vi "TTA_MATLAB_RX_Perform1RFIC1RxACPRTest.vi"(0 "Channel":string(combo), 1 "MXG VISA Resource In":refnum<visa-resource-name>, 2 "EXA VISA Resource":refnum<visa-resource-name>, 5 "Tx":string(combo), 11 "error in":errorcluster) -> (4 "ACPR\nResults":T1, 12 "MXG VISA Resource Out":refnum<visa-resource-name>, 13 "EXA VISA Resource Out":refnum<visa-resource-name>, 15 "error out":errorcluster)   [LabVIEW 2016]
uses:
  TTA_Globals/TTA_Global_Complete_Settings.vi
panel:
  out "RF Frequency":dbl[](array[numeric])
  out "ACPR Data":dbl[][](array[numeric])
  out "RFPAL PMU\nResults":dbl[][][](array[numeric])
  out "In Range?":bool[](array[boolean])
  out "Amp Max\nSpec (dBm)":dbl
  out "Amp Min\nSpec (dBm)":dbl
  out "IF Index":i32
  in  "PALLinearization Values":T2
  out "Tx#":i32
  out "CH#":i32
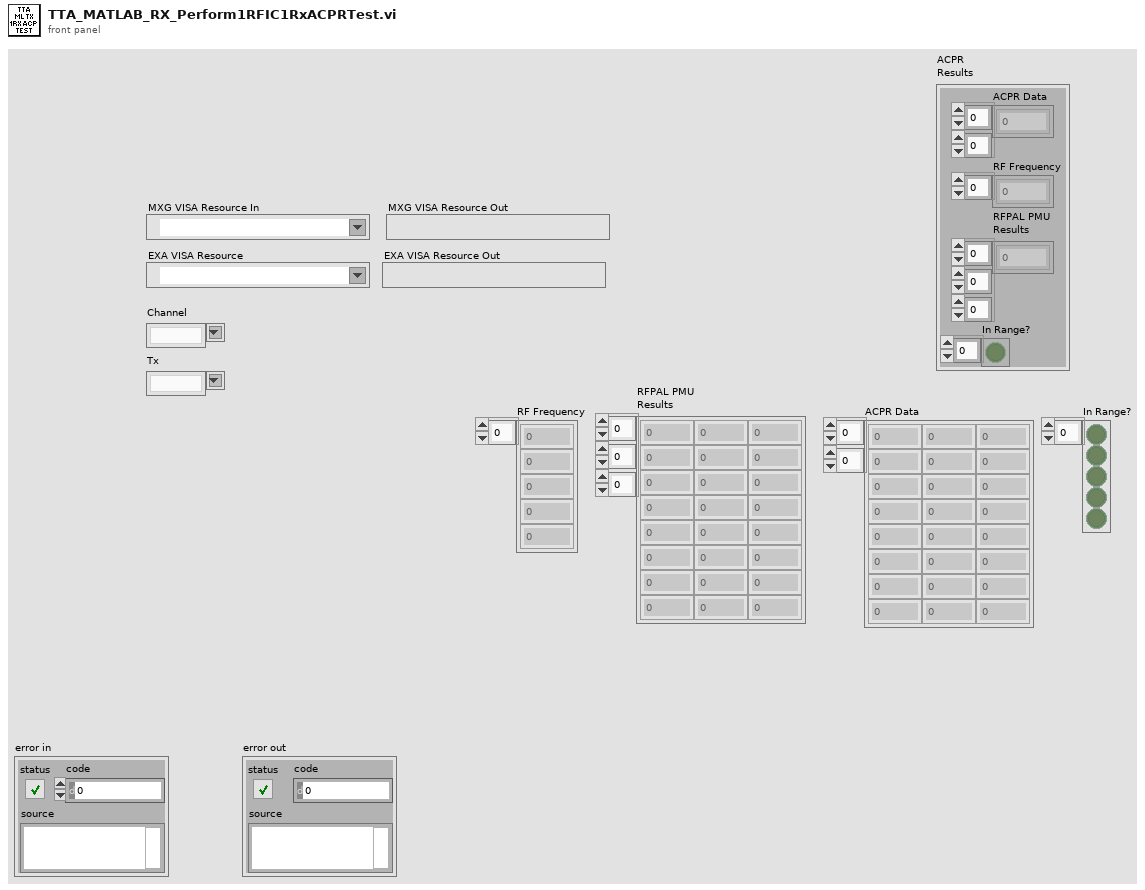
[diagram p1: front panel]
types:
  T1 = cluster{"ACPR Data":dbl[][], "RF Frequency":dbl[], "RFPAL PMU\nResults":dbl[][][], "In Range?":bool[]}
  T2 = cluster{"Tx IF Offsets":dbl[], "ACPR Filename":string, "Sampling Rate":dbl, "TxIF_Freq":dbl, "Power (dBm)":dbl, "IF Frequency Sweep (MHz)":dbl[], "BDSFreq":dbl, "Amplitude Range\nMax(dBm)":dbl, "Amplitude Range\nMin(dBm)":dbl, "CAL Amplitude\nIncrement(dB)":dbl, "CAL Amplitude\nDecrement (dB)":dbl, "Amplitude Least\nCriteria (dBm)":dbl}
  T3 = typedef "TTA_Control_Complete_Settings_Cluster.ctl" = cluster{"Brief Cluster":cluster{"STM Firmware File":string, "STM Firmware Address":string, "Required SW Version":string, "Template Used":string}, "Instrument Setting Cluster":cluster{"BDSFreq":dbl, "BDS Amp":dbl, "TxRFCal_Freq":dbl, "TxRFCal_Amp":dbl, "RxRFCal_Freq":dbl, "RxRFCal_Freq":dbl, "TxIF_Freq":dbl, "TxIF_Amp":dbl, "Tx_Output_Power_Signal_Freq":dbl, "Tx_ACPR_Signal_Freq":dbl, "Rx_RF_Freq":dbl, "Rx_RF_Amp":dbl, "Rx_Output_Power_Signal_Freq":dbl, "Rx_Output_Power_Sense_Freq":dbl}, "PAL Calibration\nInputs Cluster":cluster{"Amplitude Range\nMax(dBm)":dbl, "Amplitude Range\nMin(dBm)":dbl, "Amplitude Least\nCriteria (dBm)":dbl, "Frequency 1":dbl, "Frequency 2":dbl, "Frequency 3":dbl, "CAL Amplitude\nDecrement (dB)":dbl, "CAL Amplitude\nIncrement(dB)":dbl, "DownloadFile":string}, "TxOffset Cal Cluster":cluster{"Tx1 Offset (dB)":dbl, "Tx2 Offset (dB)":dbl, "Tx3 Offset (dB)":dbl, "Tx4 Offset (dB)":dbl, "Total RF Tx Loss (dB)":dbl}, "RxOffset Cal Cluster":cluster{"Rx1 Offset (dB)":dbl, "Rx2 Offset (dB)":dbl, "Rx3 Offset (dB)":dbl, "Rx4 Offset (dB)":dbl, "Total RF Rx Loss (dB)":dbl}, "TX Output Power Settings Cluster":cluster{"Frequency Sweep (MHz)":dbl[], "Sig Gen \nPower (dBm)":dbl, "Span (kHz)":dbl, "RBW (Hz)":dbl, "Ref Level (dBm)":dbl, "Low Power \nLimit":dbl, "High Power \nLimit":dbl, "DigAtt Max":dbl, "DigAtt Min":dbl}, "Tx ACPR Settings Cluster":cluster{"ACPR Filename":string, "Sampling Rate":dbl, "Power (dBm)":dbl, "IF Frequency Sweep (MHz)":dbl[], "State Name":string, "Mechanical\nAttenuation":dbl, "RefLevel Offset":dbl, "Amplitude Range\nMax (dBm)":dbl, "Amplitude Range\nMin (dBm)":dbl, "Cal Amp \nIncrement (dB)":dbl, "Cal Amp\nDecrement (dB)":dbl}, "Power Cal Cluster":cluster{"Power List (dBm)":dbl[], "Frequency (MHz)":dbl[], "Cal Decrement (dB)":dbl, "Cal Increment (dB)":dbl}, "Rx Received Power Settings Cluster":cluster{"Frequency Sweep (MHz)":dbl[], "Power (dBm)":dbl, "Span (kHz)":dbl, "RBW (Hz)":dbl, "Ref Level":dbl, "Low Power \nLimit (dBm)":dbl, "High Power\nLimit (dBm)":dbl}, "Tx Output Power Criteria Cluster":cluster{"CH1-TX1 \nMin":dbl, "CH1-TX1\nMax":dbl, "CH1-TXx3\nMin ":dbl, "CH1-TXx3\nMax":dbl, "CH2-TX1\nMin":dbl, "CH2-TX1\nMax":dbl, "CH2-TXx3\nMin":dbl, "CH2-TXx3\nMax":dbl}, "Tx ACPR Criteria Cluster":cluster{"Min Inband":dbl, "Max Close Outband":dbl, "Max Far Outband":dbl}, "Rx Output Power Criteria Cluster":cluster{"CH1-RX1 \nMin":dbl, "CH1-RX1 \nMax":dbl, "CH1-RXx3 \nMin":dbl, "CH1-RXx3\nMax":dbl, "CH2-RX1\nMin":dbl, "CH2-RX1\nMax":dbl, "CH2-RXx3\nMin":dbl, "CH2-RXx3\nMax":dbl}}
  T4 = cluster{"BDSFreq":dbl, "BDS Amp":dbl, "TxRFCal_Freq":dbl, "TxRFCal_Amp":dbl, "RxRFCal_Freq":dbl, "RxRFCal_Freq":dbl, "TxIF_Freq":dbl, "TxIF_Amp":dbl, "Tx_Output_Power_Signal_Freq":dbl, "Tx_ACPR_Signal_Freq":dbl, "Rx_RF_Freq":dbl, "Rx_RF_Amp":dbl, "Rx_Output_Power_Signal_Freq":dbl, "Rx_Output_Power_Sense_Freq":dbl}
  T5 = cluster{"Amplitude Range\nMax(dBm)":dbl, "Amplitude Range\nMin(dBm)":dbl, "Amplitude Least\nCriteria (dBm)":dbl, "Frequency 1":dbl, "Frequency 2":dbl, "Frequency 3":dbl, "CAL Amplitude\nDecrement (dB)":dbl, "CAL Amplitude\nIncrement(dB)":dbl, "DownloadFile":string}
  T6 = cluster{"Tx1 Offset (dB)":dbl, "Tx2 Offset (dB)":dbl, "Tx3 Offset (dB)":dbl, "Tx4 Offset (dB)":dbl, "Total RF Tx Loss (dB)":dbl}
  T7 = cluster{"ACPR Filename":string, "Sampling Rate":dbl, "Power (dBm)":dbl, "IF Frequency Sweep (MHz)":dbl[], "State Name":string, "Mechanical\nAttenuation":dbl, "RefLevel Offset":dbl, "Amplitude Range\nMax (dBm)":dbl, "Amplitude Range\nMin (dBm)":dbl, "Cal Amp \nIncrement (dB)":dbl, "Cal Amp\nDecrement (dB)":dbl}
  T8 = cluster{"CH1-TX1 \nMin":dbl, "CH1-TX1\nMax":dbl, "CH1-TXx3\nMin ":dbl, "CH1-TXx3\nMax":dbl, "CH2-TX1\nMin":dbl, "CH2-TX1\nMax":dbl, "CH2-TXx3\nMin":dbl, "CH2-TXx3\nMax":dbl}
  T9 = cluster{"Min Inband":dbl, "Max Close Outband":dbl, "Max Far Outband":dbl}
  T10 = cluster{"Amplitude Range\nMax (dBm)":dbl, "Amplitude Range\nMin (dBm)":dbl, "Cal Amp\nDecrement (dB)":dbl, "Cal Amp \nIncrement (dB)":dbl, "Amplitude Least\nCriteria (dBm)":dbl}
  T11 = enum16{"TX1", "TX2", "TX3", "TX4", "TXx3", "TXx4", "RX1", "RX2", "RX3", "RX4", "RXx3", "RXx4", "RFCal"}
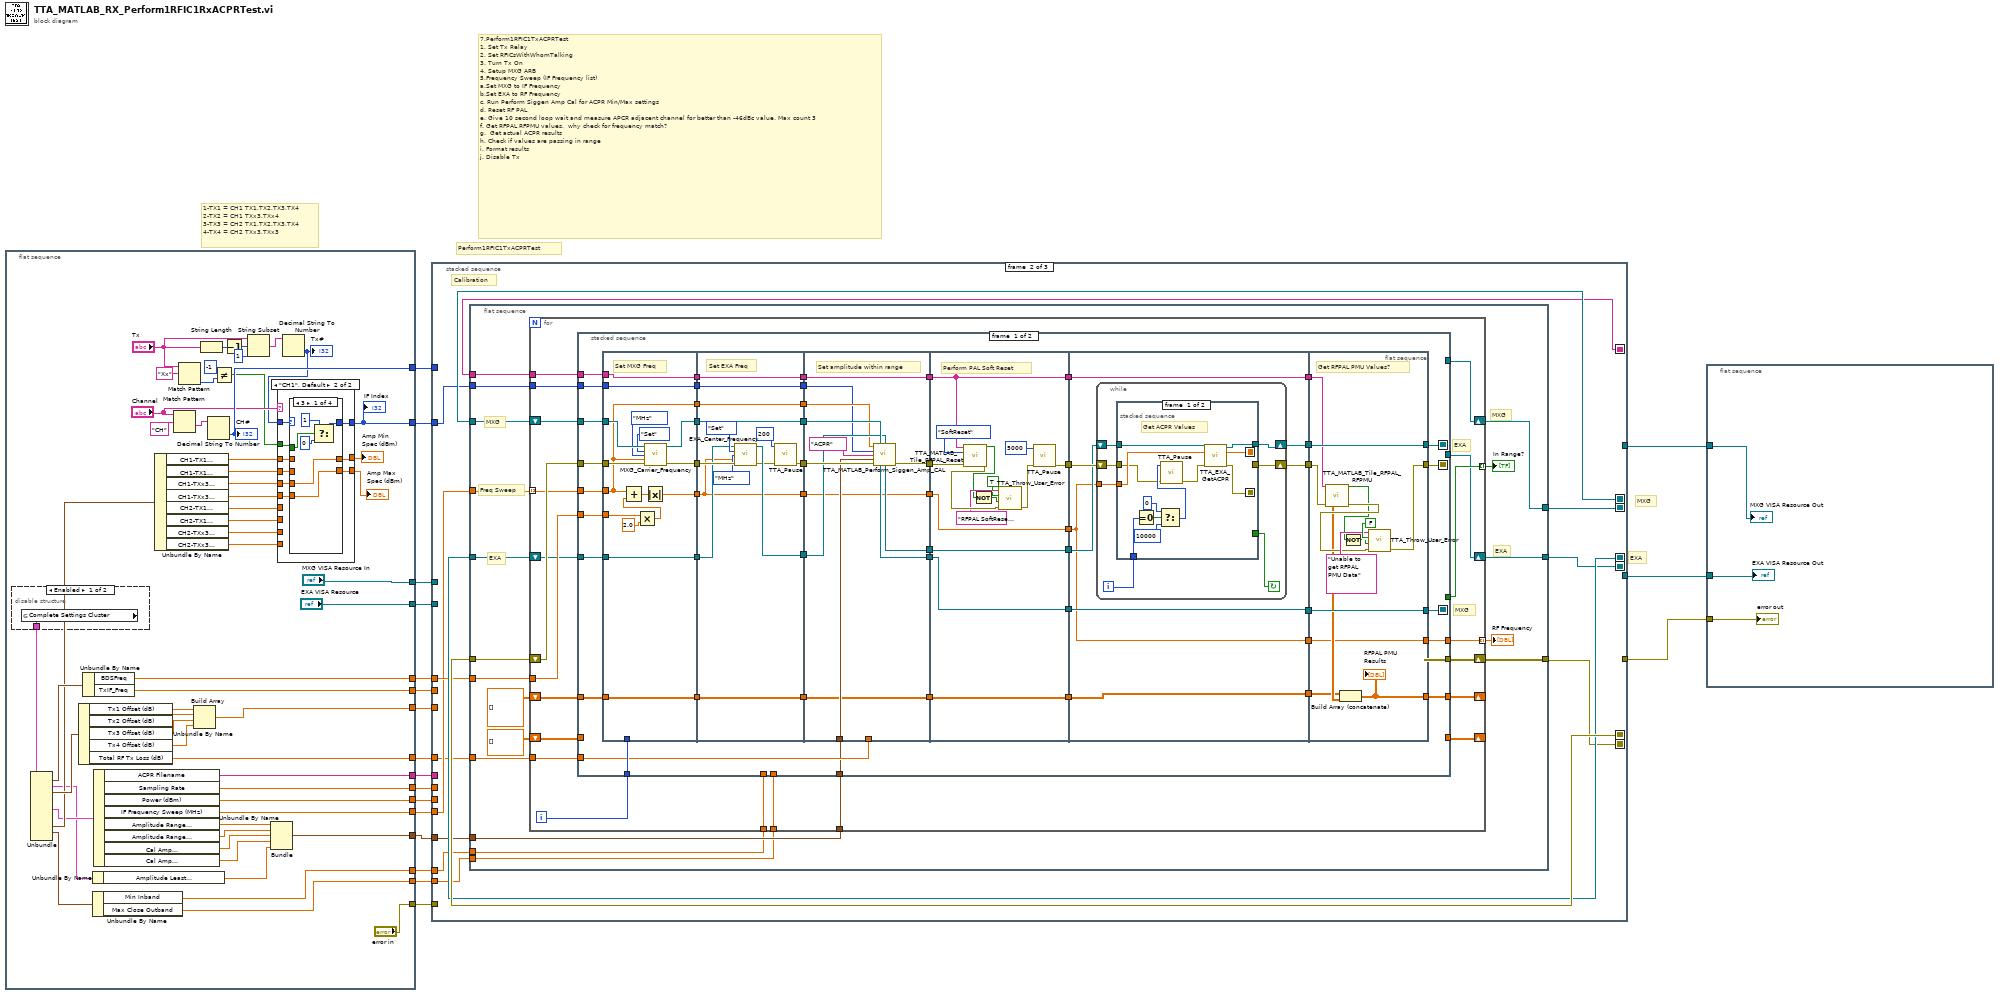
[diagram p0: block diagram]
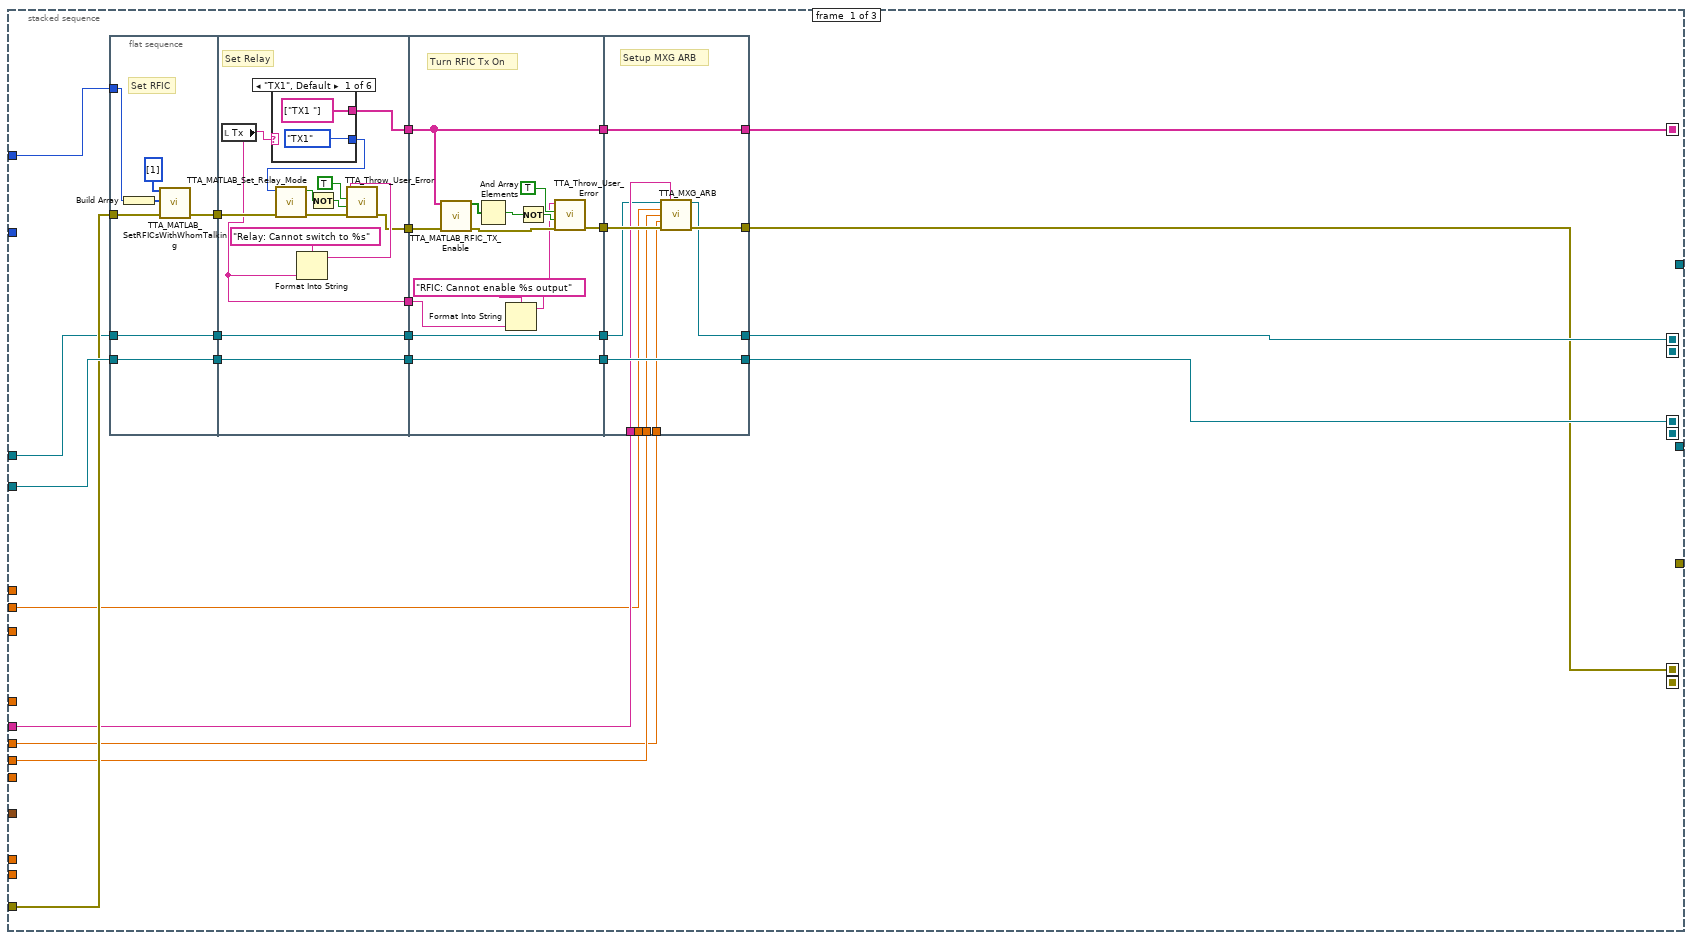
[diagram p2: hidden frame]
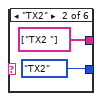
[diagram p3: hidden frame]
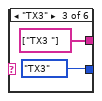
[diagram p4: hidden frame]
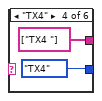
[diagram p5: hidden frame]
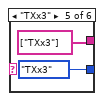
[diagram p6: hidden frame]
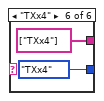
[diagram p7: hidden frame]
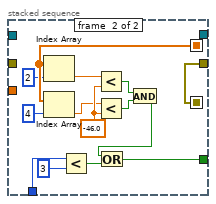
[diagram p8: hidden frame]
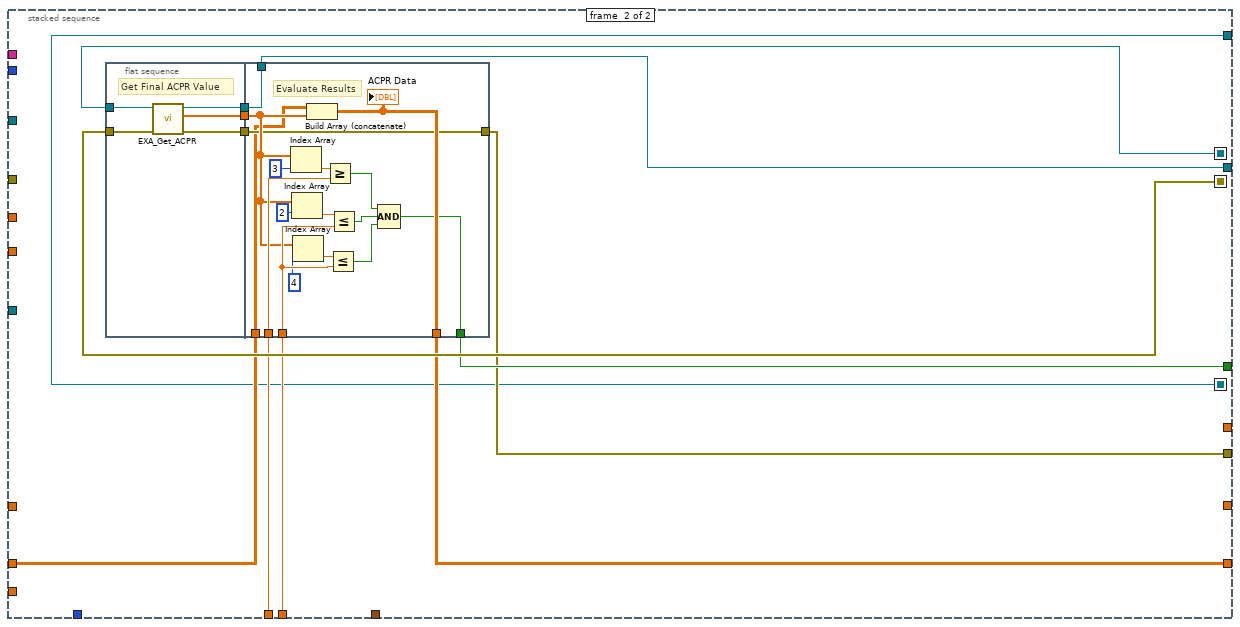
[diagram p9: hidden frame]
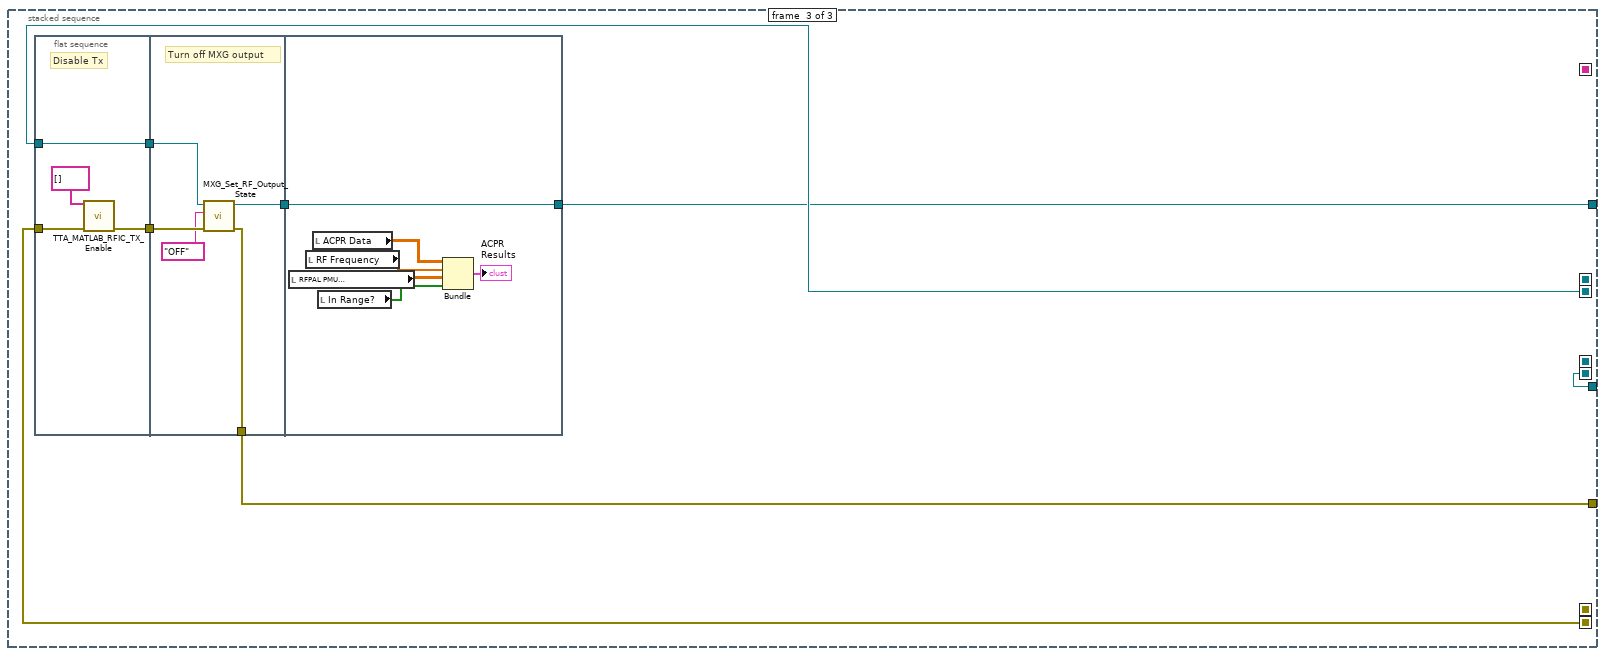
[diagram p10: hidden frame]
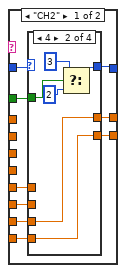
[diagram p11: hidden frame]
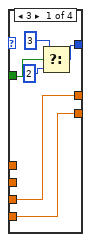
[diagram p12: hidden frame]
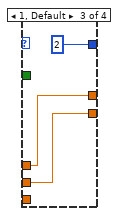
[diagram p13: hidden frame]
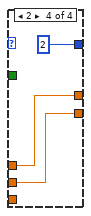
[diagram p14: hidden frame]
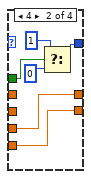
[diagram p15: hidden frame]
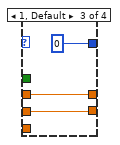
[diagram p16: hidden frame]
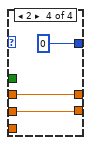
[diagram p17: hidden frame]
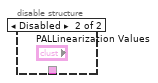
[diagram p18: hidden frame]
diagram:
  # "Perform1RFIC1TxACPRTest"
  # "7.Perform1RFIC1TxACPRTest\n1. Set Tx Relay\n2. Set RFICsWithWhomTalking\n3. Turn Tx On\n4. Setup MXG ARB\n5.Frequency Sweep (IF Frequency list)\na.Set MXG to IF Frequency\nb.Set EXA to RF Frequency\nc. Run Perform Siggen Amp Cal for ACPR Min/Max settings\nd. Reset RF PAL\ne. Give 10 second loop wait and measure APCR adjacent channel for better than -46dBc value. Max count 3\nf. Get RFPAL RFPMU values.  why check for frequency match?\ng.  Get actual ACPR results\nh. Check if values are passing in range\ni. Format results\nj. Disable Tx"
  # "1-TX1 = CH1 TX1,TX2,TX3,TX4\n2-TX2 = CH1 TXx3,TXx4\n3-TX3 = CH2 TX1,TX2,TX3,TX4\n4-TX4 = CH2 TXx3,TXx3"
  # "EXA"
  # "MXG"
  n1 = flat-sequence {
    tunnel: ["error in"] -> w19
    tunnel: ["MXG VISA Resource In"] -> w17
    tunnel: ["EXA VISA Resource"] -> w16
    tunnel: [w69] -> w18
    tunnel: [w55] -> w13
    tunnel: [w56] -> w12
    tunnel: [w61] -> w11
    tunnel: [w47] -> w10
    tunnel: [w33] -> w9
    tunnel: [w46] -> w8
    tunnel: [w32] -> w6
    tunnel: [w31] -> w5
    tunnel: [w30] -> w4
    tunnel: [w23] -> w3
    tunnel: [w21] -> w2
    tunnel: [w20] -> w1
    frame #0 {
      n2 = disable-structure shown="Enabled" {
        disable-tunnel: [w129 _] -> w64
        frame Enabled {
          n3 = global read "TTA_Global_Complete_Settings.vi" "Complete Settings Cluster"() -> (w129:T3)
        }
        frame Disabled {
        }
      }
      n4 = Unbundle(w64) -> ("Instrument Setting Cluster"=w63:T4, "PAL Calibration\nInputs Cluster"=w29:T5, "TxOffset Cal Cluster"=w62:T6, "Tx ACPR Settings Cluster"=w34:T7, "Tx Output Power Criteria Cluster"=w45:T8, "Tx ACPR Criteria Cluster"=w22:T9)  [unwired: 6 out]
      n5 = Unbundle By Name(w62) -> ("Tx1 Offset (dB)"=w60:dbl, "Tx2 Offset (dB)"=w59:dbl, "Tx3 Offset (dB)"=w58:dbl, "Tx4 Offset (dB)"=w57:dbl, "Total RF Tx Loss (dB)"=w46:dbl)
      n6 = Unbundle By Name(w63) -> ("BDSFreq"=w61:dbl, "TxIF_Freq"=w55:dbl)
      n7 = Unbundle By Name(w29) -> ("Amplitude Least\nCriteria (dBm)"=w24:dbl)
      n8 = Unbundle By Name(w22) -> ("Min Inband"=w21:dbl, "Max Close Outband"=w20:dbl)
      n9 = Unbundle By Name(w34) -> ("ACPR Filename"=w32:string, "Sampling Rate"=w30:dbl, "Power (dBm)"=w31:dbl, "IF Frequency Sweep (MHz)"=w33:dbl[], "Amplitude Range\nMax (dBm)"=w28:dbl, "Amplitude Range\nMin (dBm)"=w27:dbl, "Cal Amp\nDecrement (dB)"=w26:dbl, "Cal Amp \nIncrement (dB)"=w25:dbl)
      n10 = Unbundle By Name(w45) -> ("CH1-TX1 \nMin"=w44:dbl, "CH1-TX1\nMax"=w43:dbl, "CH1-TXx3\nMin"=w42:dbl, "CH1-TXx3\nMax"=w41:dbl, "CH2-TX1\nMin"=w40:dbl, "CH2-TX1\nMax"=w39:dbl, "CH2-TXx3\nMin"=w38:dbl, "CH2-TXx3\nMax"=w37:dbl)
      n11 = Match Pattern(string="Channel", regular expression="CH") -> (after substring=w70:string)  [unwired: 1 in, 3 out]
      n12 = Match Pattern(string="Tx", regular expression="Xx") -> (offset past match=w50:i32)  [unwired: 1 in, 3 out]
      n13 = Build Array(w60, w59, w58, w57) -> (w56:dbl[])
      n14 = String Length(string="Tx") -> (length=w68:i32)
      n15 = Decimal String To Number(string=w70) -> (number=w69:i32)  [unwired: 2 in, 1 out]
      "CH#" <- w69
      n16 = Not Equal?(x=-1, y=w50) -> (x != y?=w48:bool)
      n17 = Decrement(x=w68) -> (x-1=w67:i32)
      n18 = String Subset(string="Tx", offset (0)=w67, length (rest)=1 ("length (rest)")) -> (substring=w65:string)
      n19 = Bundle("Amplitude Range\nMax (dBm)"=w28, "Amplitude Range\nMin (dBm)"=w27, "Cal Amp\nDecrement (dB)"=w26, "Cal Amp \nIncrement (dB)"=w25, "Amplitude Least\nCriteria (dBm)"=w24) -> (w23:T10)  [unwired: 1 in]
      n20 = Decimal String To Number(string=w65) -> (number=w53:i32)  [unwired: 2 in, 1 out]
      "Tx#" <- w53
      n21 = case shown="\"CH1\", Default" "Channel" {
        tunnel: w53 -> [w82 w110]
        tunnel: [w83 w109] -> w47
        tunnel: w48 -> [w81 w108]
        tunnel: w44 -> [_ w107]
        tunnel: w43 -> [_ w106]
        tunnel: w42 -> [_ w105]
        tunnel: w41 -> [_ w104]
        tunnel: w40 -> [w80 _]
        tunnel: w39 -> [w79 _]
        tunnel: w38 -> [w78 _]
        tunnel: w37 -> [w77 _]
        tunnel: [w76 w103] -> w36
        tunnel: [w75 w102] -> w35
        frame "CH2" {
          n22 = case shown="4" w82 {
            tunnel: [w87 w93 2 2] -> w83
            tunnel: w81 -> [w86 w92 _ _]
            tunnel: w80 -> [_ _ w97 w100]
            tunnel: [w85 w91 w97 w100] -> w76
            tunnel: w79 -> [_ _ w96 w99]
            tunnel: [w84 w90 w96 w99] -> w75
            tunnel: w78 -> [w85 w91 _ _]
            tunnel: w77 -> [w84 w90 _ _]
            frame 3 {
              n23 = Select(t=3, s=w86, f=2) -> (s? t:f=w87:i32)
            }
            frame 4 {
              n24 = Select(t=3, s=w92, f=2) -> (s? t:f=w93:i32)
            }
            frame 1, Default {
            }
            frame 2 {
            }
          }
        }
        frame "CH1", Default {
          n25 = case shown="3" w110 {
            tunnel: [w114 w120 0 0] -> w109
            tunnel: w108 -> [w113 w119 _ _]
            tunnel: [w112 w118 w124 w127] -> w103
            tunnel: w107 -> [_ _ w124 w127]
            tunnel: [w111 w117 w123 w126] -> w102
            tunnel: w106 -> [_ _ w123 w126]
            tunnel: w105 -> [w112 w118 _ _]
            tunnel: w104 -> [w111 w117 _ _]
            frame 3 {
              n26 = Select(t=1, s=w113, f=0) -> (s? t:f=w114:i32)
            }
            frame 4 {
              n27 = Select(t=1, s=w119, f=0) -> (s? t:f=w120:i32)
            }
            frame 1, Default {
            }
            frame 2 {
            }
          }
        }
      }
      "IF Index" <- w47
      "Amp Min\nSpec (dBm)" <- w36
      "Amp Max\nSpec (dBm)" <- w35
    }
  }
  n28 = stacked-sequence {
    seq-local: [w130 _ _] -> [_ w222 _]
    seq-local: [w142 _ _] -> [_ w219 _]
    seq-local: [w143 _ _] -> [_ w221 _]
    seq-local: [_ w216 _] -> [_ _ w460]
    seq-local: [_ w214 _] -> [_ _ w466]
    seq-local: [_ w215 _] -> [_ _ w463]
    seq-local: [w131 _ _] -> [_ w211 _]
    tunnel: w19 -> [w141 _ _]
    tunnel: w18 -> [w153 _ _]
    tunnel: w17 -> [w140 _ _]
    tunnel: w16 -> [w151 _ _]
    tunnel: [_ _ w463] -> w15
    tunnel: [_ _ w462] -> w14
    tunnel: w13 -> [w134 _ _]
    tunnel: w12 -> [_ _ _]
    tunnel: w11 -> [_ w220 _]
    tunnel: w10 -> [_ w213 _]
    tunnel: w9 -> [_ w218 _]
    tunnel: w8 -> [_ w217 _]
    tunnel: [_ _ w464] -> w7
    tunnel: w6 -> [w135 _ _]
    tunnel: w5 -> [w133 _ _]
    tunnel: w4 -> [w132 _ _]
    tunnel: w3 -> [_ w212 _]
    tunnel: w2 -> [_ w210 _]
    tunnel: w1 -> [_ w209 _]
    frame #0 {
      n29 = flat-sequence {
        tunnel: [w157] -> w152
        tunnel: [w154] -> w150
        tunnel: [w156] -> w149
        tunnel: w153 -> [w158]
        tunnel: w151 -> [w156]
        tunnel: w141 -> [w155]
        tunnel: w140 -> [w154]
        tunnel: w152 -> [w173]
        tunnel: w150 -> [w165]
        tunnel: w149 -> [w163]
        tunnel: [w165] -> w148
        tunnel: [w161] -> w147
        tunnel: [w164] -> w146
        tunnel: [w163] -> w145
        tunnel: [w162] -> w144
        tunnel: w148 -> [w187]
        tunnel: w147 -> [w191]
        tunnel: w146 -> [w190]
        tunnel: w145 -> [w189]
        tunnel: w144 -> [w188]
        tunnel: [w189] -> w139
        tunnel: [w191] -> w138
        tunnel: [w187] -> w137
        tunnel: [w186] -> w136
        tunnel: [w199] -> w142
        tunnel: [w207] -> w131
        tunnel: [w208] -> w143
        tunnel: w139 -> [w208]
        tunnel: w138 -> [w207]
        tunnel: w137 -> [w204]
        tunnel: w136 -> [w206]
        tunnel: w135 -> [w205]
        tunnel: w134 -> [w203]
        tunnel: w133 -> [w202]
        tunnel: w132 -> [w201]
        tunnel: [w200] -> w130
        frame #0 {
          # "Set RFIC"
          n30 = Build Array(w158) -> (w159:i32[])
          n31 = call "TTA_MATLAB_SetRFICsWithWhomTalking.vi"("Panel Array"=i32[] [1], "RFIC Array"=w159, "error in"=w155) -> ("error out"=w157:errorcluster)  [unwired: 12 in]
        }
        frame #1 {
          # "Set Relay"
          n32 = local read "Tx"() -> (w162:string)
          n33 = case shown="\"TX1\", Default" w162 {
            tunnel: [T11."TX1" ("Mode") T11."TX2" ("Mode") T11."TX3" ("Mode") T11."TX4" ("Mode") T11."TXx3" ("Mode") T11."TXx4" ("Mode")] -> w172
            tunnel: [string[] ["TX1 "] ("Channels") string[] ["TX2 "] ("Channels") string[] ["TX3 "] ("Channels") string[] ["TX4 "] ("Channels") string[] ["TXx3"] ("Channels") string[] ["TXx4"] ("Channels")] -> w161
            frame "TX1", Default {
            }
            frame "TX2" {
            }
            frame "TX3" {
            }
            frame "TX4" {
            }
            frame "TXx3" {
            }
            frame "TXx4" {
            }
          }
          n34 = call "TTA_MATLAB_Set_Relay_Mode.vi"("error in"=w173, "Mode"=w172) -> ("error out"=w171:errorcluster, "Success"=w170:bool)  [unwired: 8 in]
          n35 = Format Into String(format string="Relay: Cannot switch to %s", w162) -> (resulting string=w166:string)  [unwired: 2 in, 1 out]
          n36 = Not(x=w170) -> (.not. x?=w169:bool)
          n37 = call "TTA_Throw_User_Error.vi"("error in"=w171, "Error?"=w169, "Stop Execution on Fail"=TRUE, "Error Message"=w166) -> ("error out"=w164:errorcluster)  [unwired: 7 in]
        }
        frame #2 {
          # "Turn RFIC Tx On"
          n38 = call "TTA_MATLAB_RFIC_TX_Enable.vi"("Channels"=w191, "error in"=w190) -> ("SuccessComm"=w198:bool[], "error out"=w194:errorcluster)  [unwired: 12 in]
          n39 = And Array Elements(Boolean array=w198) -> (logical AND=w195:bool)
          n40 = Format Into String(format string="RFIC: Cannot enable %s output", w188) -> (resulting string=w192:string)  [unwired: 2 in, 1 out]
          n41 = Not(x=w195) -> (.not. x?=w196:bool)
          n42 = call "TTA_Throw_User_Error.vi"("error in"=w194, "Error?"=w196, "Stop Execution on Fail"=TRUE, "Error Message"=w192) -> ("error out"=w186:errorcluster)  [unwired: 7 in]
        }
        frame #3 {
          # "Setup MXG ARB"
          n43 = call "TTA_MXG_ARB.vi"("VISA resource In"=w204, "Waveform File"=w205, "Frequency (MHz)"=w203, "Output Power\nLevel (dBm)"=w202, "ARB Sample Rate"=w201, "error in"=w206) -> ("VISA resource Out"=w199:refnum<visa-resource-name>, "error out"=w200:errorcluster)  [unwired: 8 in]
        }
      }
    }
    frame #1 {
      # "Calibration"
      n44 = flat-sequence {
        tunnel: w222 -> [w240]
        tunnel: w221 -> [w239]
        tunnel: [w238] -> w215
        tunnel: [w237] -> w216
        tunnel: w220 -> [w236]
        tunnel: w218 -> [w235]
        tunnel: w219 -> [w234]
        tunnel: w217 -> [w233]
        tunnel: [w232] -> w214
        tunnel: w213 -> [w230]
        tunnel: w212 -> [w229]
        tunnel: w211 -> [w228]
        tunnel: w210 -> [w226]
        tunnel: w209 -> [w225]
        frame #0 {
          # "EXA"
          # "MXG"
          # "Freq Sweep"
          # "EXA"
          # "MXG"
          n45 = for {
            shift-right: [w244] -> w237
            shift-left: w240 -> [w258]
            shift-right: [w243] -> w238
            shift-left: w239 -> [w257]
            tunnel: w236 -> [w260]
            tunnel: w235 -> [w256] mode=indexing
            shift-right: [w241] -> w232
            shift-left: w234 -> [w259]
            tunnel: w233 -> [w255]
            tunnel: [w246] -> w231 mode=indexing
            tunnel: w230 -> [w254]
            tunnel: w229 -> [w253]
            tunnel: w228 -> [w252]
            shift-right: [w251] -> _
            shift-left: dbl[][][] [] -> [w250]
            tunnel: w226 -> [w249]
            tunnel: w225 -> [w248]
            shift-right: [w247] -> _
            shift-left: dbl[][] [] -> [w242]
            tunnel: [w245] -> w224 mode=indexing
            i -> [w261]
            # "EXA"
            # "MXG"
            n46 = stacked-sequence {
              seq-local: [w278 _] -> [_ w436]
              seq-local: [w275 _] -> [_ w425]
              seq-local: [w273 _] -> [_ w437]
              tunnel: w261 -> [w289 _]
              tunnel: w260 -> [w288 _]
              tunnel: w259 -> [w287 _]
              tunnel: w258 -> [w286 _]
              tunnel: w257 -> [w285 _]
              tunnel: w256 -> [w284 _]
              tunnel: w255 -> [w283 _]
              tunnel: w254 -> [w282 _]
              tunnel: w253 -> [w281 _]
              tunnel: w252 -> [w280 _]
              tunnel: [w270 _] -> w251
              tunnel: w250 -> [w269 _]
              tunnel: w249 -> [_ w432]
              tunnel: w248 -> [_ w431]
              tunnel: [_ w430] -> w247
              tunnel: [_ w429] -> w246
              tunnel: [w262 _] -> w245
              tunnel: [_ w428] -> w244
              tunnel: [_ w427] -> w243
              tunnel: w242 -> [_ w426]
              tunnel: [_ w425] -> w241
              frame #0 {
                n47 = flat-sequence {
                  tunnel: w284 -> [w315]
                  tunnel: w289 -> [_]
                  tunnel: w288 -> [w323]
                  tunnel: w287 -> [w326]
                  tunnel: w286 -> [w327]
                  tunnel: w285 -> [w317]
                  tunnel: [w319] -> w311
                  tunnel: [w318] -> w310
                  tunnel: [w317] -> w309
                  tunnel: [w316] -> w308
                  tunnel: [w315] -> w307
                  tunnel: w282 -> [w314]
                  tunnel: [w314] -> w306
                  tunnel: w280 -> [w313]
                  tunnel: [w313] -> w305
                  tunnel: w269 -> [w312]
                  tunnel: [w312] -> w268
                  tunnel: w311 -> [w329]
                  tunnel: w310 -> [w341]
                  tunnel: w309 -> [w339]
                  tunnel: w308 -> [w336]
                  tunnel: [w337] -> w304
                  tunnel: [w336] -> w303
                  tunnel: [w333] -> w302
                  tunnel: [w332] -> w301
                  tunnel: w307 -> [w332]
                  tunnel: [w331] -> w300
                  tunnel: w306 -> [w331]
                  tunnel: [w330] -> w299
                  tunnel: w305 -> [w330]
                  tunnel: [w329] -> w298
                  tunnel: w268 -> [w328]
                  tunnel: [w328] -> w267
                  tunnel: w304 -> [w351]
                  tunnel: w303 -> [w352]
                  tunnel: w302 -> [w354]
                  tunnel: w283 -> [_]
                  tunnel: w301 -> [w350]
                  tunnel: w300 -> [w349]
                  tunnel: w281 -> [w348]
                  tunnel: [w347] -> w297
                  tunnel: [w346] -> w296
                  tunnel: w299 -> [w346]
                  tunnel: [w345] -> w295
                  tunnel: [w344] -> w294
                  tunnel: w298 -> [w343]
                  tunnel: [w343] -> w293
                  tunnel: w267 -> [w342]
                  tunnel: [w342] -> w266
                  tunnel: w297 -> [w363]
                  tunnel: w296 -> [w356]
                  tunnel: w295 -> [w357]
                  tunnel: w294 -> [w358]
                  tunnel: [w361] -> w292
                  tunnel: w293 -> [w359]
                  tunnel: [w359] -> w291
                  tunnel: [w358] -> w290
                  tunnel: [w357] -> w277
                  tunnel: [w356] -> w271
                  tunnel: w266 -> [w355]
                  tunnel: [w355] -> w265
                  tunnel: w292 -> [w377]
                  tunnel: w291 -> [w370]
                  tunnel: w290 -> [w376]
                  tunnel: [w375] -> w279
                  tunnel: w277 -> [w374]
                  tunnel: [w374] -> w276
                  tunnel: [w373] -> w274
                  tunnel: [w372] -> w272
                  tunnel: w271 -> [w372]
                  tunnel: w265 -> [w371]
                  tunnel: [w371] -> w264
                  tunnel: [w370] -> w263
                  tunnel: w279 -> [w424]
                  tunnel: [w424] -> w278
                  tunnel: w276 -> [w423]
                  tunnel: [w423] -> w275
                  tunnel: w274 -> [w422]
                  tunnel: [w415] -> w273
                  tunnel: w272 -> [w421]
                  tunnel: [w413] -> w270
                  tunnel: w264 -> [w412]
                  tunnel: w263 -> [w411]
                  tunnel: [w411] -> w262
                  frame #0 {
                    # "Set MXG Freq"
                    n48 = Multiply(x=w323, y=2.0) -> (x*y=w321:dbl)
                    n49 = Add(x=w315, y=w321) -> (x+y=w320:dbl)
                    n50 = Absolute Value(x=w320) -> (abs(x)=w319:dbl)
                    n51 = call "MXG_Carrier_Frequency.vi"("VISA resource name"=w326, "Mode"=enum16{"Set", "Get"}."Set", "Units"=enum16{"Hz", "kHz", "MHz", "GHz"}."MHz", "Frequency"=w315, "error in"=w327) -> ("VISA resource name"=w316:refnum<visa-resource-name>, "error out"=w318:errorcluster)  [unwired: 8 in, 1 out]
                  }
                  frame #1 {
                    # "Set EXA Freq"
                    n52 = call "EXA_Center_Frequency.vi"("VISA resource name"=w339, "Mode"=enum16{"Set", "Get"}."Set", "Units"=enum16{"Hz", "kHz", "MHz", "GHz"}."MHz", "Frequency"=w329, "error in"=w341) -> ("VISA resource name"=w337:refnum<visa-resource-name>, "error out"=w335:errorcluster)  [unwired: 8 in, 1 out]
                    n53 = call "TTA_Pause.vi"("error in"=w335, "Pause (ms)"=u32 200) -> ("error out"=w333:errorcluster)  [unwired: 9 in]
                  }
                  frame #2 {
                    # "Set amplitude within range"
                    n54 = call "TTA_MATLAB_Perform_Siggen_Amp_CAL.vi"("IF Frequency (MHz)"=w350, "MXG VISA Resource In"=w352, "EXA VISA Resource"=w351, "IF Index"=w349, "Test"="ACPR", "Amp CAL Criteria Cluster"=w348, "error in"=w354) -> ("MXG VISA Resource Out"=w345:refnum<visa-resource-name>, "EXA VISA Resource Out"=w344:refnum<visa-resource-name>, "error out"=w347:errorcluster)  [unwired: 4 in, 2 out]
                  }
                  frame #3 {
                    # "Perform PAL Soft Reset"
                    n55 = call "TTA_MATLAB_Tile_RFPAL_Reset.vi"("Channels"=w356, "Mode"=enum16{"SoftReset", "HardReset"}."SoftReset", "error in"=w363) -> ("Success"=w367:bool, "error out"=w369:errorcluster)  [unwired: 9 in, 2 out]
                    n56 = Not(x=w367) -> (.not. x?=w366:bool)
                    n57 = call "TTA_Throw_User_Error.vi"("error in"=w369, "Error?"=w366, "Stop Execution on Fail"=TRUE, "Error Message"="RFPAL SoftReset not successful") -> ("error out"=w362:errorcluster)  [unwired: 7 in]
                    n58 = call "TTA_Pause.vi"("error in"=w362, "Pause (ms)"=u32 5000) -> ("error out"=w361:errorcluster)  [unwired: 9 in]
                  }
                  frame #4 {
                    n59 = while {
                      shift-right: [w378] -> w373
                      shift-left: w377 -> [w384]
                      tunnel: w370 -> [w383]
                      shift-right: [w380] -> w375
                      shift-left: w376 -> [w382]
                      i -> [w381]
                      stop <- w379 continue-if-true
                      n60 = stacked-sequence {
                        seq-local: [w393 _] -> [_ w407]
                        seq-local: [w386 _] -> [_ w397]
                        tunnel: w384 -> [w388 _]
                        tunnel: w383 -> [w396 _]
                        tunnel: w382 -> [w395 _]
                        tunnel: w381 -> [w392 w410]
                        tunnel: [w385 _] -> w380
                        tunnel: [_ w398] -> w379
                        tunnel: [_ w397] -> w378
                        frame #0 {
                          # "Get ACPR Values"
                          n61 = Equal To 0?(x=w392) -> (x = 0?=w391:bool)
                          n62 = Select(t=0, s=w391, f=10000) -> (s? t:f=w389:i32)
                          n63 = call "TTA_Pause.vi"("error in"=w388, "Pause (ms)"=w389) -> ("error out"=w394:errorcluster)  [unwired: 9 in]
                          n64 = call "TTA_EXA_GetACPR.vi"("VISA resource In"=w395, "Frequency (MHz)"=w396, "error in"=w394) -> ("VISA resource Out"=w385:refnum<visa-resource-name>, "ACP Values"=w393:dbl[], "error out"=w386:errorcluster)  [unwired: 10 in]
                        }
                        frame #1 {
                          w404 = -46.0
                          n65 = Index Array(array=w407, index=2) -> (element=w403:dbl)
                          n66 = Index Array(array=w407, index=4) -> (element=w402:dbl)
                          n67 = Less?(x=w410, y=3) -> (x < y?=w408:bool)
                          n68 = Less?(x=w403, y=w404) -> (x < y?=w400:bool)
                          n69 = Less?(x=w402, y=w404) -> (x < y?=w401:bool)
                          n70 = And(x=w400, y=w401) -> (x .and. y?=w399:bool)
                          n71 = Or(x=w399, y=w408) -> (x .or. y?=w398:bool)
                        }
                      }
                    }
                  }
                  frame #5 {
                    # "Get RFPAL PMU Values?"
                    n72 = call "TTA_MATLAB_Tile_RFPAL_RFPMU.vi"("Channels"=w421, "error in"=w422) -> ("Success"=w416:bool, "Tile Outputs"=w414:dbl[][], "error out"=w417:errorcluster)  [unwired: 9 in, 2 out]
                    n73 = Build Array (concatenate)(w412, w414) -> (w413:dbl[][][])
                    "RFPAL PMU\nResults" <- w413
                    n74 = Not(x=w416) -> (.not. x?=w419:bool)
                    n75 = call "TTA_Throw_User_Error.vi"("error in"=w417, "Error?"=w419, "Stop Execution on Fail"=FALSE, "Error Message"="Unable to get RFPAL PMU Data") -> ("error out"=w415:errorcluster)  [unwired: 7 in]
                  }
                }
              }
              frame #1 {
                n76 = flat-sequence {
                  tunnel: w437 -> [w442]
                  tunnel: w436 -> [w441]
                  tunnel: [w440] -> w435
                  tunnel: [w439] -> w434
                  tunnel: [w438] -> w433
                  tunnel: w435 -> [w452]
                  tunnel: w434 -> [w444]
                  tunnel: w433 -> [w445]
                  tunnel: w432 -> [w457]
                  tunnel: w431 -> [w456]
                  tunnel: [w447] -> w430
                  tunnel: [w446] -> w429
                  tunnel: [w445] -> w427
                  tunnel: [w444] -> w428
                  tunnel: w426 -> [w443]
                  frame #0 {
                    # "Get Final ACPR Value"
                    n77 = call "EXA_Get_ACPR.vi"("error in"=w442, "VISA resource name"=w441) -> ("error out"=w439:errorcluster, "ACP Values"=w440:dbl[], "VISA resource name"=w438:refnum<visa-resource-name>)  [unwired: 7 in]
                  }
                  frame #1 {
                    # "Evaluate Results"
                    n78 = Index Array(array=w452, index=3) -> (element=w458:dbl)
                    n79 = Index Array(array=w452, index=2) -> (element=w451:dbl)
                    n80 = Index Array(array=w452, index=4) -> (element=w455:dbl)
                    n81 = Build Array (concatenate)(w443, w452) -> (w447:dbl[][])
                    "ACPR Data" <- w447
                    n82 = Greater Or Equal?(x=w458, y=w457) -> (x >= y?=w450:bool)
                    n83 = Less Or Equal?(x=w455, y=w456) -> (x <= y?=w448:bool)
                    n84 = Less Or Equal?(x=w451, y=w456) -> (x <= y?=w449:bool)
                    n85 = Compound Arithmetic op=AND(w450, w449, w448) -> (w446:bool)
                  }
                }
              }
            }
          }
          "In Range?" <- w231
          "RF Frequency" <- w224
        }
      }
    }
    frame #2 {
      n86 = flat-sequence {
        tunnel: [w470] -> w467
        tunnel: [w469] -> w465
        tunnel: w466 -> [w469]
        tunnel: w460 -> [w468]
        tunnel: w467 -> [w476]
        tunnel: w465 -> [w475]
        tunnel: [w472] -> w462
        tunnel: [w473] -> w461
        tunnel: [w482] -> w464
        tunnel: w461 -> [w482]
        frame #0 {
          # "Disable Tx"
          n87 = call "TTA_MATLAB_RFIC_TX_Enable.vi"("Channels"=string[] [], "error in"=w468) -> ("error out"=w470:errorcluster)  [unwired: 12 in, 1 out]
        }
        frame #1 {
          # "Turn off MXG output"
          n88 = call "MXG_Set_RF_Output_State.vi"("error in"=w476, "RF Output State"="OFF", "VISA resource name"=w475) -> ("error out"=w472:errorcluster, "VISA resource name"=w473:refnum<visa-resource-name>)  [unwired: 7 in]
        }
        frame #2 {
          n89 = local read "RFPAL PMU\nResults"() -> (w479:dbl[][][])
          n90 = local read "RF Frequency"() -> (w480:dbl[])
          n91 = local read "ACPR Data"() -> (w481:dbl[][])
          n92 = local read "In Range?"() -> (w478:bool[])
          n93 = Bundle("ACPR Data"=w481, "RF Frequency"=w480, "RFPAL PMU\nResults"=w479, "In Range?"=w478) -> (→"ACPR\nResults":T1)  [unwired: 1 in]
        }
      }
    }
  }
  n94 = flat-sequence {
    tunnel: w15 -> [w485]
    tunnel: w14 -> [w484]
    tunnel: w7 -> [w483]
    frame #0 {
      "error out" <- w484
      "MXG VISA Resource Out" <- w483
      "EXA VISA Resource Out" <- w485
    }
  }
